vi "Selected Doc Name[].vi"(8 "error in (no error)":errorcluster, 11 "ListBox in":refnum<vi>) -> (0 "error out":errorcluster, 3 "Array":string[](array[string]))   [LabVIEW 2016]
doc: "Returns selected Document Names in array"
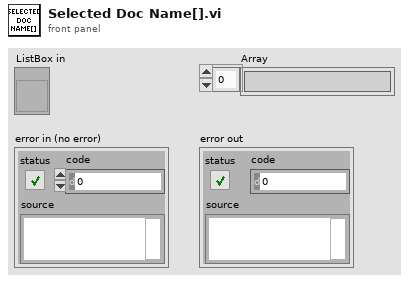
[diagram p1: front panel]
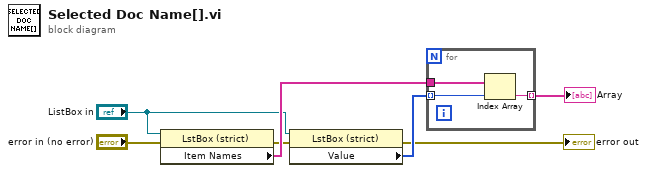
[diagram p0: block diagram]
diagram:
  n1 = property on="Property Node" class="LstBox (strict)"(reference="ListBox in", error in="error in (no error)") -> (error out=w5:errorcluster, "Item Names"=w6:string[])  [unwired: 1 out]
  n2 = property on="Property Node" class="LstBox (strict)"(reference="ListBox in", error in=w5) -> (error out=→"error out":errorcluster, "Value"=w4:i32[])  [unwired: 1 out]
  n3 = for {
    tunnel: w6 -> [w10]
    tunnel: w4 -> [w9] mode=indexing
    tunnel: [w8] -> w7 mode=indexing
    n4 = Index Array(array=w10, index=w9) -> (element=w8:string)
  }
  "Array" <- w7
